vi "EGT_SubVI.vi"(0 "High Byte":u8, 3 "Low Byte":u8) -> (7 "EGT":u16)   [LabVIEW 2012]
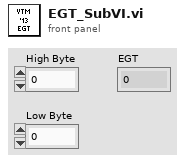
[diagram p1: front panel]
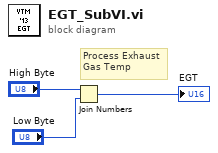
[diagram p0: block diagram]
diagram:
  # "Process Exhaust\nGas Temp"
  n1 = Join Numbers(hi="High Byte", lo="Low Byte") -> ((hi.lo)=→"EGT":u16)
